vi "Integer Definition.vi"(11 "Integer in":refnum<class "Integer.lvclass">) -> (2 "Definition":T1)   [LabVIEW 2020, in "Conditu2.lvlib" / "Columns.lvlib" / "Integer.lvclass"]
uses:
  Integer.lvclass
  Definition.ctl
  Integer.lvclass/Integer.ctl
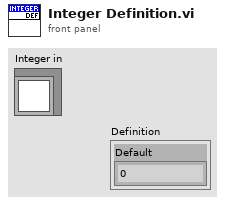
[diagram p1: front panel]
types:
  T1 = typedef "Conditu2.lvlib/Columns.lvlib/Integer.lvclass/Definition.ctl" = cluster{"Default":i64}
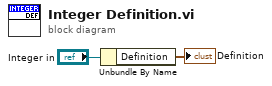
[diagram p0: block diagram]
diagram:
  n1 = Unbundle By Name("Integer in") -> ("Definition"=→"Definition":T1)
